vi "usbpt104UnitInfo.vi"(8 "error in (no error)":errorcluster, 11 "handle in":i16=16384) -> (0 "error out":errorcluster, 2 "Unit Info":T1, 3 "handle out":i16=16384)   [LabVIEW 2010]
doc: "Returns Driver and Unit Information"
uses:
  UsbPT104.dll
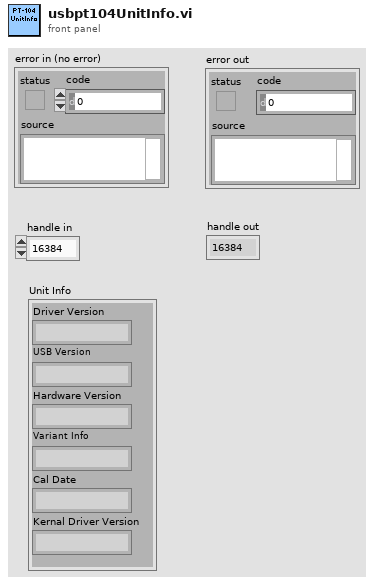
[diagram p1: front panel]
types:
  T1 = cluster{"Driver Version":string, "USB Version":string, "Hardware Version":string, "Variant Info":string, "Cal Date":string, "Kernal Driver Version":string, "NA":string, "NA 2":string, "NA":string, "NA 3":string, "NA 4":string, "NA 5":string, "NA 6":string, "NA 7":string, "NA 8":string}
  T2 = cluster{"[0]":string, "[1]":string, "[2]":string, "[3]":string, "[4]":string, "[5]":string, "[6]":string, "[7]":string, "[8]":string, "[9]":string, "[10]":string, "[11]":string, "[12]":string, "[13]":string, "[14]":string}
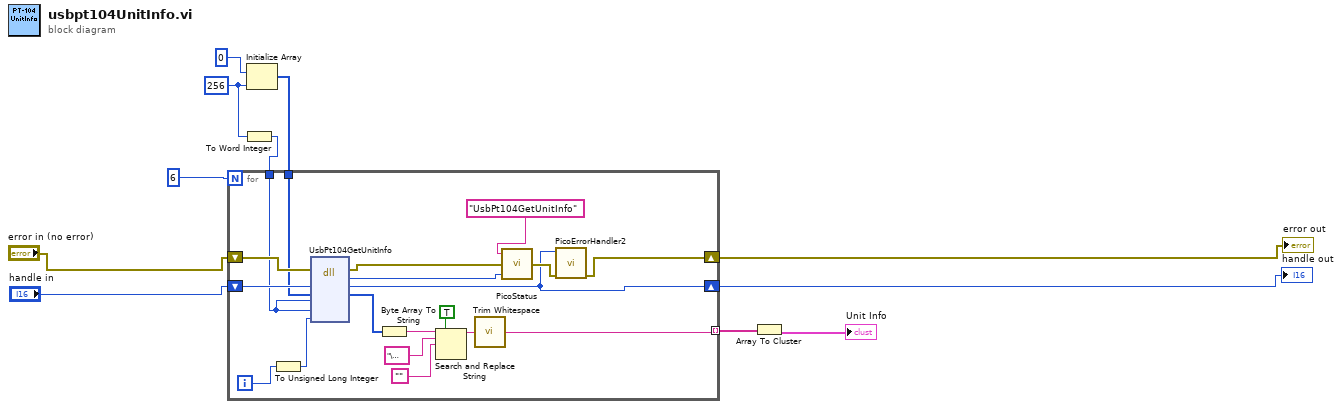
[diagram p0: block diagram]
diagram:
  w5 = 256 ("dimension size")
  n1 = To Word Integer(number=w5) -> (16bit integer=w4:i16)
  n2 = Initialize Array(u8 0 ("element"), w5) -> (w11:u8[])
  n3 = for {
    N: 6 -> [_]
    tunnel: [w13] -> w8 mode=indexing
    tunnel: w11 -> [w24]
    shift-right: [w14] -> w2
    shift-left: "handle in" -> [w26]
    shift-right: [w16] -> w3
    shift-left: "error in (no error)" -> [w25]
    tunnel: w4 -> [w12]
    i -> [w20]
    n4 = To Unsigned Long Integer(number=w20) -> (unsigned 32bit integer=w21:u32)
    n5 = dll-call lib="UsbPT104.dll" fn="UsbPt104GetUnitInfo"(error in=w25, "handle"=w26, "String"=w24, "StringLength"=w12, "requiredSize"=w12, "info"=w21) -> (error out=w17:errorcluster, "PICO_STATUS"=w15:u32, "handle"=w14:i16, "String"=w23:u8[])  [unwired: 5 in, 1 out]
    n6 = Byte Array To String(unsigned byte array=w23) -> (string=w22:string)
    n7 = Search and Replace String(replace all?=TRUE ("replace all? (F)"), input string=w22, search string="\u0000", replace string="") -> (result string=w27:string)  [unwired: 4 in, 3 out]
    n8 = call <vilib>:"Trim Whitespace.vi"("string"=w27) -> ("trimmed string"=w13:string)  [unwired: 1 in]
    n9 = call "PicoStatus.vi"("PICO STATUS"=w15, "error in"=w17, "source"="UsbPt104GetUnitInfo") -> ("error out"=w19:errorcluster)
    n10 = call "PicoErrorHandler2.vi"("error in (no error)"=w19, "handle In"=w14) -> ("error out"=w16:errorcluster)  [unwired: 9 in]
  }
  "error out" <- w3
  "handle out" <- w2
  n11 = Array To Cluster(array=w8) -> (cluster=→"Unit Info":T2)
